vi "ReadUncertainties.vi"(7 "error in (no error)":errorcluster) -> (0 "error out":errorcluster, 3 "Uncertainties":dbl[][][](array[numeric]) format="%#_4g")   [LabVIEW 2014]
uses:
  Excel(ActiveX)/enumOpenOrCreate.ctl
  Excel(ActiveX)/Excel(ActiveX).lvlib
panel:
  # "VA TVE"
  # "VB TVE"
  # "VC TVE"
  # "V+ TVE"
  # "IA TVE"
  # "IB TVE"
  # "IC TVE"
  # "I+ TVE"
  # "Freq Hz"
  # "ROCOF HZ/s"
  # "FreqRng"
  # "MagRng"
  # "Harmonics"
  # "Out-of-Band"
  # "Phase Mod"
  # "Amplitude Mod"
  # "FreqRamp +"
  # "FreqRamp -"
  # "Phase Step Pos"
  # "Phase Step Pos Mag"
  # "Phase Step Pos Phase"
  # "Phase Step Neg"
  # "Phase Step Neg Mag"
  # "Phase Step Neg Phase"
  # "Mag Step Pos"
  # "Mag Step Pos Mag"
  # "Mag Step Pos Phase"
  # "Mag Step Neg"
  # "Mag Step Neg Mag"
  # "Mag Step Neg Phase"
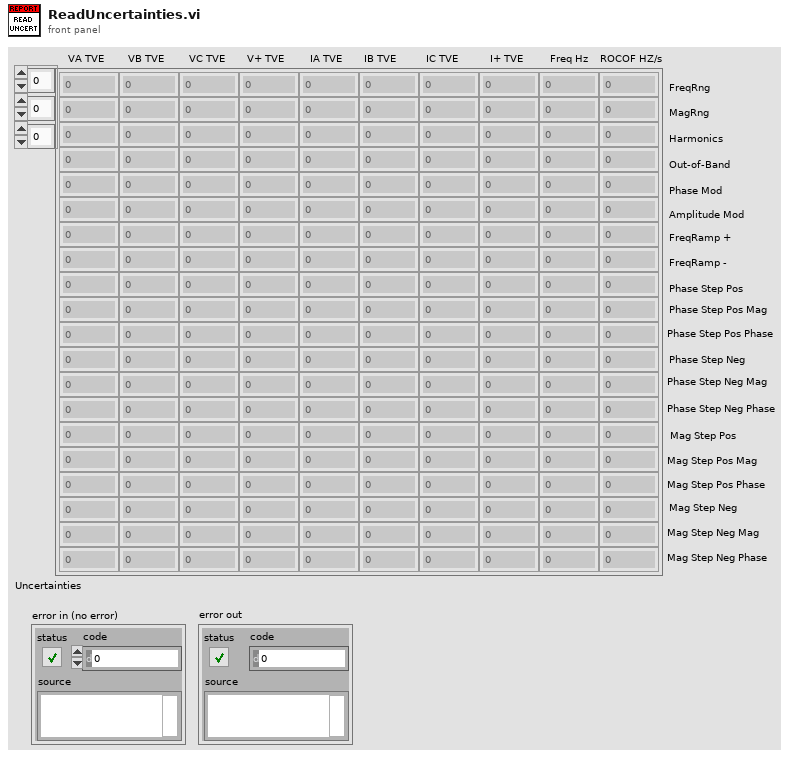
[diagram p1: front panel]
types:
  T1 = typedef "Excel(ActiveX).lvlib/enumOpenOrCreate.ctl" = enum16{"open", "open or create", "create from template"}
  T2 = typedef "Excel(ActiveX).lvlib/ExcelActiveX.ctl" = cluster{"Excel._Application":refnum<k7>, "Application open at start":bool, "Excel._Worksheet":refnum<k7>, "Workbook open at start":bool, "Excel._Workbook":refnum<k7>, "Workbook Path":path, "Worksheet Name":string, "Row":u32, "Col":u32, "Cell":string, "Workbook Name":string}
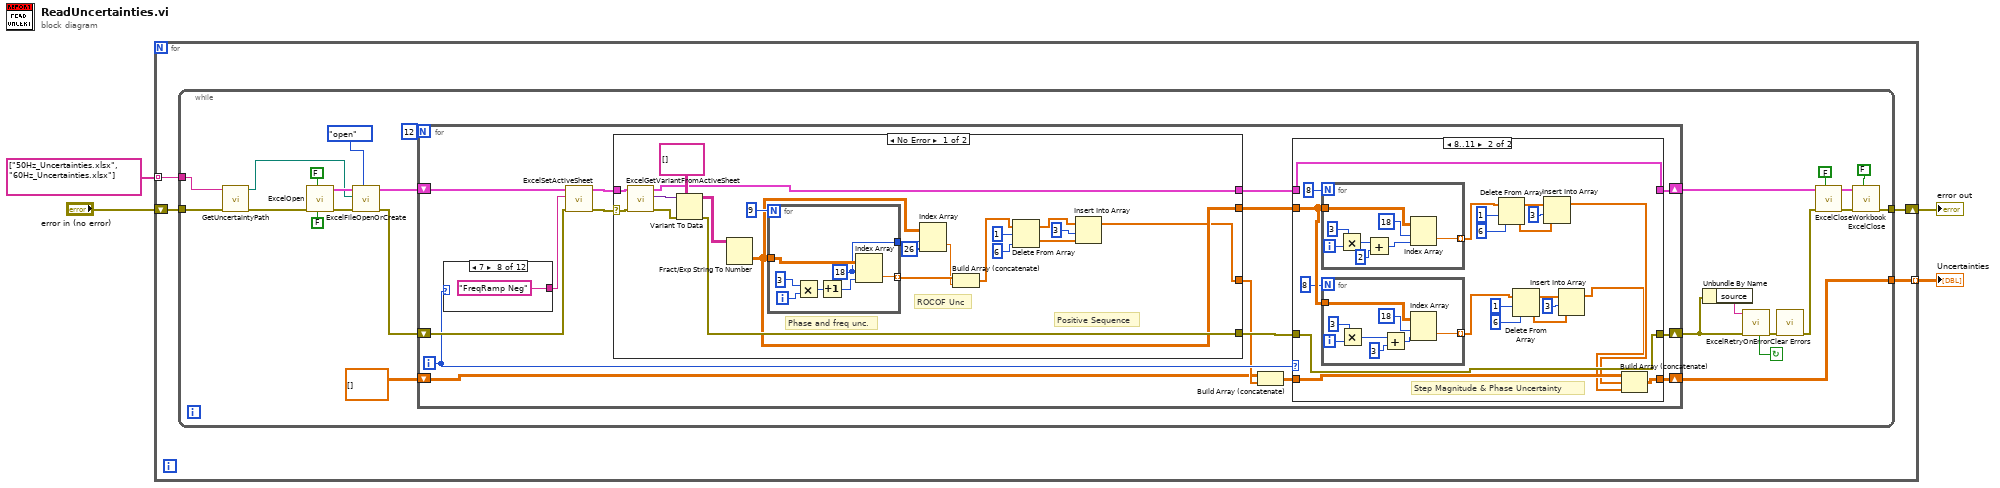
[diagram p0: block diagram]
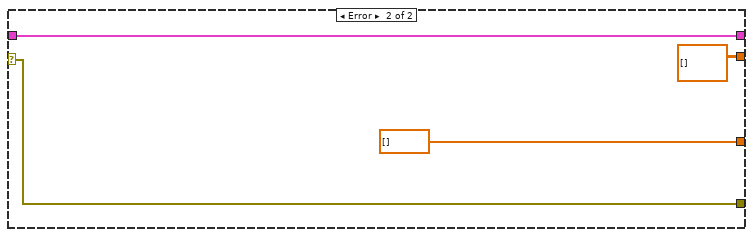
[diagram p3: hidden frame]
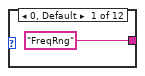
[diagram p4: hidden frame]
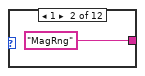
[diagram p5: hidden frame]
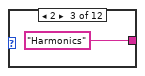
[diagram p6: hidden frame]
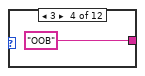
[diagram p7: hidden frame]
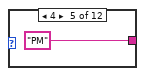
[diagram p8: hidden frame]
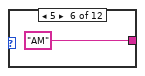
[diagram p9: hidden frame]
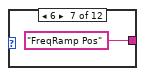
[diagram p10: hidden frame]
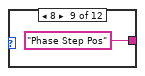
[diagram p11: hidden frame]
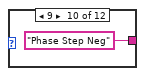
[diagram p12: hidden frame]
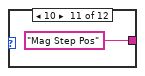
[diagram p13: hidden frame]
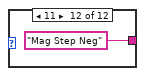
[diagram p14: hidden frame]
diagram:
  n1 = for {
    shift-right: [w7] -> w3
    shift-left: "error in (no error)" -> [w8]
    tunnel: string[] ["50Hz_Uncertainties.xlsx", "60Hz_Uncertainties.xlsx"] -> [w6] mode=indexing
    tunnel: [w5] -> w1 mode=indexing
    n2 = while {
      tunnel: [w21] -> w5
      tunnel: w8 -> [w14]
      tunnel: [w32] -> w7
      tunnel: w6 -> [w12]
      stop <- w25 continue-if-true
      n3 = call "GetUncertaintyPath.vi"("error in (no error)"=w14, "FileName"=w12) -> ("error out"=w13:errorcluster, "Path"=w11:path)  [unwired: 8 in]
      n4 = call "ExcelOpen.vi"("Run Minimized (f)"=FALSE, "Excel visible? (t)"=FALSE, "error in (no error)"=w13) -> ("error out"=w10:errorcluster, "ExcelActiveX"=w28:T2)  [unwired: 7 in]
      n5 = call "ExcelFileOpenOrCreate.vi"("Open or Create"=enumOpenOrCreate."open", "error in (no error)"=w10, "Excel file name and path"=w11, "ExcelActiveX in"=w28) -> ("error out"=w30:errorcluster, "ExcelActiveX out"=w29:T2)  [unwired: 6 in]
      n6 = for {
        N: 12 -> [_]
        shift-right: [w39] -> w19
        shift-left: w29 -> [w48]
        shift-right: [w42] -> w24
        shift-left: w30 -> [w47]
        shift-right: [w35] -> w21
        shift-left: dbl[][] [] -> [w34]
        i -> [w41]
        n7 = case shown="7" w41 {
          tunnel: ["FreqRng" "MagRng" "Harmonics" "OOB" "PM" "AM" "FreqRamp Pos" "FreqRamp Neg" "Phase Step Pos" "Phase Step Neg" "Mag Step Pos" "Mag Step Neg"] -> w46
          frame 0, Default {
          }
          frame 1 {
          }
          frame 2 {
          }
          frame 3 {
          }
          frame 4 {
          }
          frame 5 {
          }
          frame 6 {
          }
          frame 7 {
          }
          frame 8 {
          }
          frame 9 {
          }
          frame 10 {
          }
          frame 11 {
          }
        }
        n8 = call "ExcelSetActiveSheet.vi"("error in (no error)"=w47, "Sheet Name"=w46, "ExcelActiveX in"=w48) -> ("error out"=w44:errorcluster, "ExcelActiveX  out"=w45:T2)  [unwired: 7 in]
        n9 = case shown="No Error" w44 {
          selector: w44 -> [w98 w119]
          tunnel: w45 -> [w109 w120]
          tunnel: [w105 w120] -> w40
          tunnel: [w89 dbl[] []] -> w37
          tunnel: [w99 w119] -> w43
          tunnel: [w95 dbl[][] []] -> w38
          frame No Error {
            # "Positive Sequence"
            # "ROCOF Unc"
            # "Phase and freq unc."
            n10 = call "ExcelGetVariantFromActiveSheet.vi"("error in (no error)"=w98, "ExcelActiveX  in"=w109) -> ("error out"=w108:errorcluster, "VariantOut"=w106:variant, "ExcelActiveX  out"=w105:T2)  [unwired: 7 in]
            n11 = Variant To Data(error in=w108, type=string[][] [], Variant=w106) -> (data=w96:string[][], error out=w99:errorcluster)
            n12 = Fract/Exp String To Number(string=w96) -> (number=w95:dbl[][])  [unwired: 3 in, 1 out]
            n13 = for {
              N: 9 -> [_]
              tunnel: w95 -> [w113]
              tunnel: [w115] -> w103 mode=indexing
              tunnel: [w112] -> w102
              i -> [w111]
              w112 = 18 ("disabled index (row)")
              n14 = Multiply(x=3, y=w111) -> (x*y=w114:i32)
              n15 = Increment(x=w114) -> (x+1=w110:i32)
              n16 = Index Array(array=w113, index (row)=w112, index (col)=w110) -> (element=w115:dbl)
            }
            n17 = Index Array(array=w95, index (row)=w102, index (col)=26 ("disabled index (col)")) -> (element=w100:dbl)
            n18 = Build Array (concatenate)(w103, w100) -> (w92:dbl[])
            n19 = Delete From Array(array=w92, length=1, index=6) -> (deleted portion=w93:dbl[], array with subset deleted=w90:dbl[])
            n20 = Insert Into Array(array=w90, index=3, new element=w93) -> (w89:dbl[])
          }
          frame Error {
          }
        }
        n21 = Build Array (concatenate)(w34, w37) -> (w36:dbl[][])
        n22 = case shown="8..11" w41 {
          tunnel: [w51 w68] -> w42
          tunnel: w43 -> [w51 w68]
          tunnel: w40 -> [w50 w72]
          tunnel: [w50 w72] -> w39
          tunnel: w38 -> [_ w69]
          tunnel: [w49 w70] -> w35
          tunnel: w36 -> [w49 w71]
          frame 0, Default {
          }
          frame 8..11 {
            # "Step Magnitude & Phase Uncertainty"
            n23 = for {
              N: 8 -> [_]
              tunnel: w69 -> [w86]
              tunnel: [w85] -> w63 mode=indexing
              i -> [w84]
              n24 = Multiply(x=3, y=w84) -> (x*y=w83:i32)
              n25 = Add(x=w83, y=2) -> (x+y=w81:i32)
              n26 = Index Array(array=w86, index (row)=18, index (col)=w81) -> (element=w85:dbl)
            }
            n27 = for {
              N: 8 -> [_]
              tunnel: w69 -> [w77]
              tunnel: [w76] -> w53 mode=indexing
              i -> [w73]
              n28 = Multiply(x=3, y=w73) -> (x*y=w75:i32)
              n29 = Add(x=w75, y=3) -> (x+y=w79:i32)
              n30 = Index Array(array=w77, index (row)=18, index (col)=w79) -> (element=w76:dbl)
            }
            n31 = Delete From Array(array=w63, length=1 ("index"), index=6) -> (deleted portion=w61:dbl[], array with subset deleted=w62:dbl[])
            n32 = Delete From Array(array=w53, length=1 ("index"), index=6) -> (deleted portion=w57:dbl[], array with subset deleted=w56:dbl[])
            n33 = Insert Into Array(array=w62, index=3, new element=w61) -> (w59:dbl[])
            n34 = Insert Into Array(array=w56, index=3, new element=w57) -> (w52:dbl[])
            n35 = Build Array (concatenate)(w71, w59, w52) -> (w70:dbl[][])
          }
        }
      }
      n36 = Unbundle By Name(w24) -> ("source"=w23:string)
      n37 = call "ExcelRetryOnError.vi"("error in (no error)"=w24, "Error Msg"=w23) -> ("error out"=w22:errorcluster, "Retry"=w25:bool)  [unwired: 8 in]
      n38 = call <vilib>:"Clear Errors.vi"("error in (no error)"=w22) -> ("error out"=w16:errorcluster)  [unwired: 5 in, 1 out]
      n39 = call "ExcelCloseWorkbook.vi"("Save"=FALSE, "error in (no error)"=w16, "ExcelActiveX"=w19) -> ("error out"=w15:errorcluster, "ExcelActiveX"=w18:T2)  [unwired: 7 in]
      n40 = call "ExcelClose.vi"("Leave Open (f)"=FALSE, "error in (no error)"=w15, "ExcelActiveX in"=w18) -> ("error out"=w32:errorcluster)  [unwired: 7 in, 1 out]
    }
  }
  "Uncertainties" <- w1
  "error out" <- w3
